vi "WriteValue_Control1.vi"(9 "value":T1, 11 "reference":refnum<vi>) -> ()   [LabVIEW 2012]
uses:
  Typedefs/Control 1.ctl
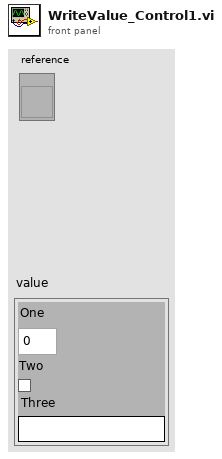
[diagram p1: front panel]
types:
  T1 = typedef "Control 1.ctl" = cluster{"One":dbl, "Two":bool, "Three":string}
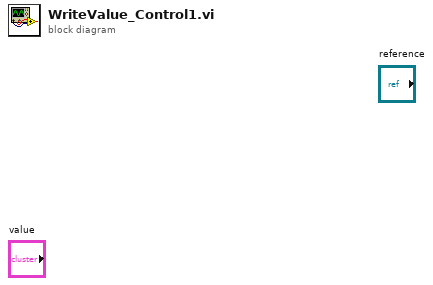
[diagram p0: block diagram]
diagram:
